vi "handleTimeout.vi"(8 "error in (no error)":errorcluster) -> (0 "error out":errorcluster)   [LabVIEW 2012]
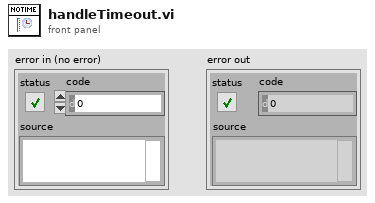
[diagram p1: front panel]
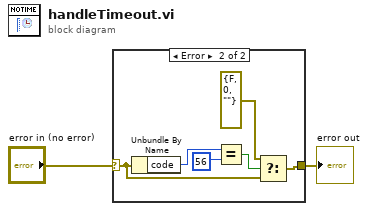
[diagram p0: block diagram]
diagram:
  n1 = case shown="Error" "error in (no error)" {
    selector: "error in (no error)" -> [w3 w4]
    tunnel: [w3 w7] -> w1
    frame No Error {
    }
    frame Error {
      n2 = Unbundle By Name(w4) -> ("code"=w9:i32)
      n3 = Equal?(x=w9, y=56) -> (x = y?=w8:bool)
      n4 = Select(t=errorcluster {"status"=FALSE, "code"=0, "source"=""} ("error out 2"), s=w8, f=w4) -> (s? t:f=w7:errorcluster)
    }
  }
  "error out" <- w1
